vi "validate configuration.vi"(8 "error in":errorcluster, 11 "TDMS datalogger configuration in":refnum<class "TDMS datalogger configuration.lvclass">) -> (0 "error out":errorcluster, 3 "TDMS datalogger configuration out":refnum<class "TDMS datalogger configuration.lvclass">)   [LabVIEW 2013, in "TDMS datalogger configuration.lvclass"]
doc: "This function performs validation of the configuration. This function should be safe to call at any point and should not rely on anything in the runtime environment."
uses:
  TDMS datalogger configuration.lvclass
  TDMS datalogger configuration.lvclass/TDMS datalogger configuration.ctl
  <vilib>/NI/Tag Bus Module Framework/module configuration/TBM module configuration.lvclass
  Read Path.vi
  Read backup directory.vi
  <vilib>/NI/Tag Bus Module Framework/root configuration/TBM configuration.lvclass
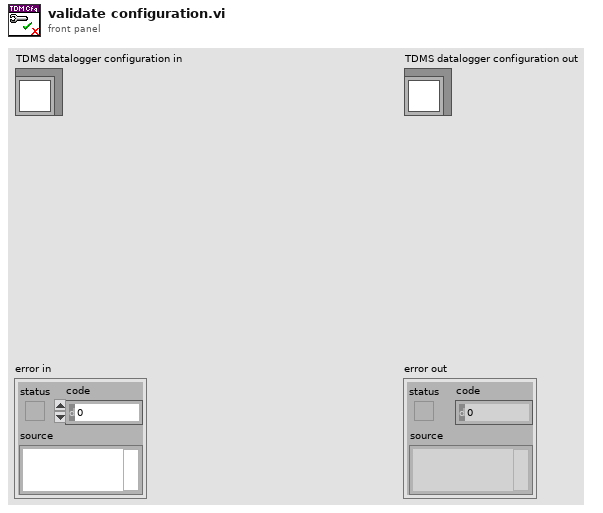
[diagram p1: front panel]
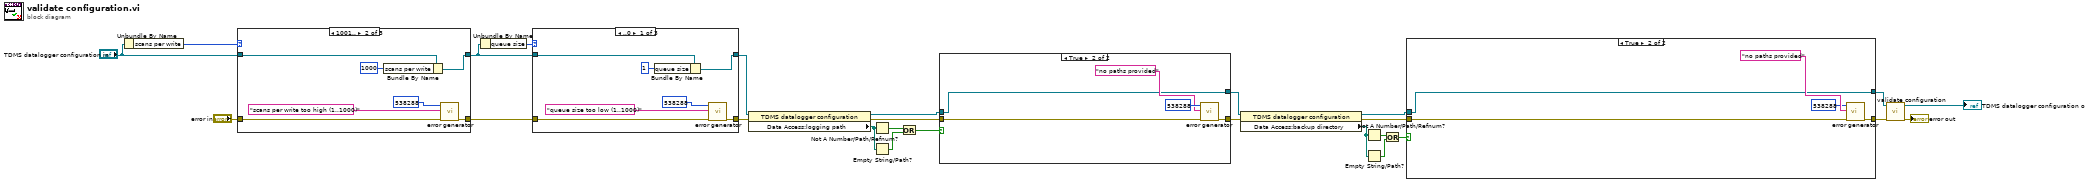
[diagram p0: block diagram]
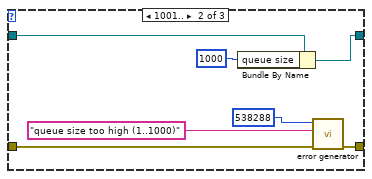
[diagram p3: hidden frame]
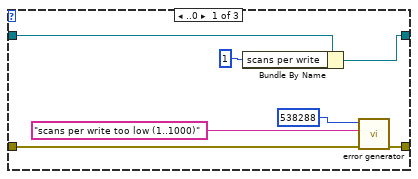
[diagram p5: hidden frame]
diagram:
  n1 = Unbundle By Name("TDMS datalogger configuration in") -> ("scans per write"=w22:i32)
  n2 = case shown="1001.." w22 {
    tunnel: [w29 w36 w42] -> w21
    tunnel: "TDMS datalogger configuration in" -> [w30 w37 w42]
    tunnel: [w31 w38 w41] -> w20
    tunnel: "error in" -> [w32 w39 w41]
    frame ..0 {
      n3 = Bundle By Name(cluster=w30, "scans per write"=1) -> (w29:refnum<class "TDMS datalogger configuration.lvclass">)
      n4 = call <vilib>:"error generator.vi"("error in"=w32, "append error message"="scans per write too low (1..1000)" ("error message (\"\")"), "error code (0)"=538288) -> ("error out"=w31:errorcluster)  [unwired: 8 in]
    }
    frame 1001.. {
      n5 = Bundle By Name(cluster=w37, "scans per write"=1000) -> (w36:refnum<class "TDMS datalogger configuration.lvclass">)
      n6 = call <vilib>:"error generator.vi"("error in"=w39, "append error message"="scans per write too high (1..1000)" ("error message (\"\")"), "error code (0)"=538288) -> ("error out"=w38:errorcluster)  [unwired: 8 in]
    }
    frame 1..1000 {
    }
  }
  n7 = Unbundle By Name(w21) -> ("queue size"=w19:i32)
  n8 = case shown="..0" w19 {
    tunnel: [w45 w52 w58] -> w13
    tunnel: w21 -> [w46 w53 w58]
    tunnel: [w47 w54 w57] -> w18
    tunnel: w20 -> [w48 w55 w57]
    frame ..0 {
      n9 = Bundle By Name(cluster=w46, "queue size"=1 ("scans per write")) -> (w45:refnum<class "TDMS datalogger configuration.lvclass">)
      n10 = call <vilib>:"error generator.vi"("error in"=w48, "append error message"="queue size too low (1..1000)" ("error message (\"\")"), "error code (0)"=538288) -> ("error out"=w47:errorcluster)  [unwired: 8 in]
    }
    frame 1001.. {
      n11 = Bundle By Name(cluster=w53, "queue size"=1000 ("scans per write")) -> (w52:refnum<class "TDMS datalogger configuration.lvclass">)
      n12 = call <vilib>:"error generator.vi"("error in"=w55, "append error message"="queue size too high (1..1000)" ("error message (\"\")"), "error code (0)"=538288) -> ("error out"=w54:errorcluster)  [unwired: 8 in]
    }
    frame 1..1000 {
    }
  }
  n13 = property class="TDMS datalogger configuration"(reference=w13, error in=w18) -> (reference out=w12:refnum<class "TDMS datalogger configuration.lvclass">, error out=w14:errorcluster, "Data Access:logging path"=w1:path)
  n14 = Not A Number/Path/Refnum?(number/path/refnum=w1) -> (NaN/Path/Refnum?=w25:bool)
  n15 = Empty String/Path?(string/path=w1) -> (empty?=w24:bool)
  n16 = Or(x=w25, y=w24) -> (x .or. y?=w23:bool)
  n17 = case shown="True" w23 {
    tunnel: [w60 w64] -> w15
    tunnel: w14 -> [w60 w62]
    tunnel: [w59 w61] -> w10
    tunnel: w12 -> [w59 w61]
    frame False {
    }
    frame True {
      n18 = call <vilib>:"error generator.vi"("error in"=w62, "append error message"="no paths provided" ("error message (\"\")"), "error code (0)"=538288) -> ("error out"=w64:errorcluster)  [unwired: 8 in]
    }
  }
  n19 = property class="TDMS datalogger configuration"(reference=w10, error in=w15) -> (reference out=w5:refnum<class "TDMS datalogger configuration.lvclass">, error out=w3:errorcluster, "Data Access:backup directory"=w2:path)
  n20 = Not A Number/Path/Refnum?(number/path/refnum=w2) -> (NaN/Path/Refnum?=w8:bool)
  n21 = Empty String/Path?(string/path=w2) -> (empty?=w9:bool)
  n22 = Or(x=w8, y=w9) -> (x .or. y?=w7:bool)
  n23 = case shown="True" w7 {
    tunnel: [w67 w69] -> w6
    tunnel: w5 -> [w67 w69]
    tunnel: [w66 w70] -> w4
    tunnel: w3 -> [w66 w68]
    frame False {
    }
    frame True {
      n24 = call <vilib>:"error generator.vi"("error in"=w68, "append error message"="no paths provided" ("error message (\"\")"), "error code (0)"=538288) -> ("error out"=w70:errorcluster)  [unwired: 8 in]
    }
  }
  n25 = call-parent "validate configuration.vi"("error in"=w4, "configuration in"=w6) -> ("error out"=→"error out":errorcluster, "configuration out"=→"TDMS datalogger configuration out":refnum<class "TDMS datalogger configuration.lvclass">)  [unwired: 8 in]
